vi "Main.vi"(11 "Module Admin":refnum<class "Delacor_lib_QMH_Module Admin.lvclass">) -> ()   [LabVIEW 2024, in "Explore.lvlib"]
doc: "This template is based off of the Queued Message Handler design pattern and the Queued Message Handler project template that ships with LabVIEW.\n\nThe main difference is that the queue is private to this module and communication between modules is performed via Broadcast and Request events.\n\nRequest events are wrapped in public API methods and are handled in the Event Handling Loop (EHL) of this VI. Any module can register for Broadcast events sent by this module. The EHL generates messages based on user interface actions.\n\nThe Message Handling Loop (MHL) processes messages generated by the EHL, or by other messages. The messages are string values, so new messages can be added easily to the Message Cases case structure in the MHL. Each message cluster can also provide an optional value for Message Data, which is a variant that can be converted to whatever message-specific data is required.\n_____\nBased on DQMH Project Template 7.0.1.1316."
uses:
  Explore.lvlib
  <vilib>/Delacor/Delacor QMH/Libraries/Module Admin_class/Delacor_lib_QMH_Module Admin.lvclass
  Module Data--cluster.ctl
  <vilib>/Delacor/Delacor QMH/Libraries/Message Queue_class/Delacor_lib_QMH_Message Queue.lvclass/Delacor_lib_QMH_Message Queue.ctl
  Stop Argument--cluster.ctl
  <vilib>/Delacor/Delacor QMH/Libraries/Module Admin_class/Delacor_lib_QMH_Module Admin.lvclass/Delacor_lib_QMH_Module Admin.ctl
  Update Table Argument--cluster.ctl
  Delete File Argument--cluster.ctl
  Get Reference Argument--cluster.ctl
  Get Reference (Reply Payload)--cluster.ctl
  <vilib>/Delacor/Delacor QMH/Libraries/Message Queue_class/Delacor_lib_QMH_Enqueue Message (Single).vi
  <vilib>/Delacor/Delacor QMH/Libraries/Module Admin_class/Delacor_lib_QMH_Get External Launch.vi
  <vilib>/Delacor/Delacor QMH/Libraries/Message Queue_class/Delacor_lib_QMH_Message Queue.lvclass
panel:
  in  "File List":i32(listbox)
  in  "Delete":bool
  out "error out":errorcluster
  out "Status":string
  in  "Simulate MHL Error":bool
  in  "Simulate EHL Error":bool
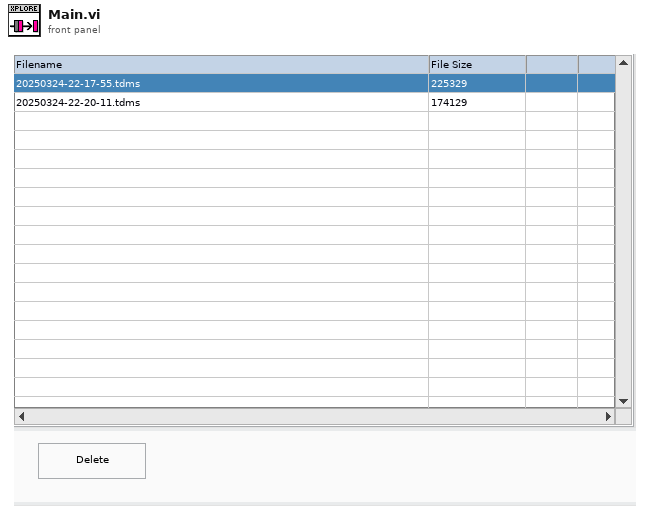
[diagram p1: front panel]
types:
  T1 = typedef "Explore.lvlib/Request Events--cluster.ctl" = cluster{"Stop Module":refnum<user-event>, "Show Panel":refnum<user-event>, "Hide Panel":refnum<user-event>, "Get Module Execution Status":refnum<user-event>, "Show Diagram":refnum<user-event>, "Update Table":refnum<user-event>, "Delete File":refnum<user-event>, "Get Reference":refnum<user-event>}
  T2 = typedef "Explore.lvlib/Module Data--cluster.ctl" = cluster{"Status":string, "Current Path":path}
  T3 = enum32{"invalid lock state", "Not Locked", "Locked (No Password)", "Password-protected"}
  T4 = typedef "Explore.lvlib/Stop Argument--cluster.ctl" = cluster{"Origin":string, "Exit via Stop Module Req?":bool, "Wait for Module to stop?":bool}
  T5 = typedef "Explore.lvlib/Update Table Argument--cluster.ctl" = cluster{"Log Folder":path}
  T6 = typedef "Explore.lvlib/Delete File Argument--cluster.ctl" = cluster{"File Name":string}
  T7 = typedef "Explore.lvlib/Get Reference Argument--cluster.ctl" = cluster{"Wait Notifier":refnum<notifier>, "wait for reply":bool}
  T8 = enum32{"Invalid", "Standard", "Closed", "Hidden", "Minimized", "Maximized"}
  T9 = typedef "Explore.lvlib/Get Reference (Reply Payload)--cluster.ctl" = cluster{"VI Refnum":refnum<vi>, "error":errorcluster}
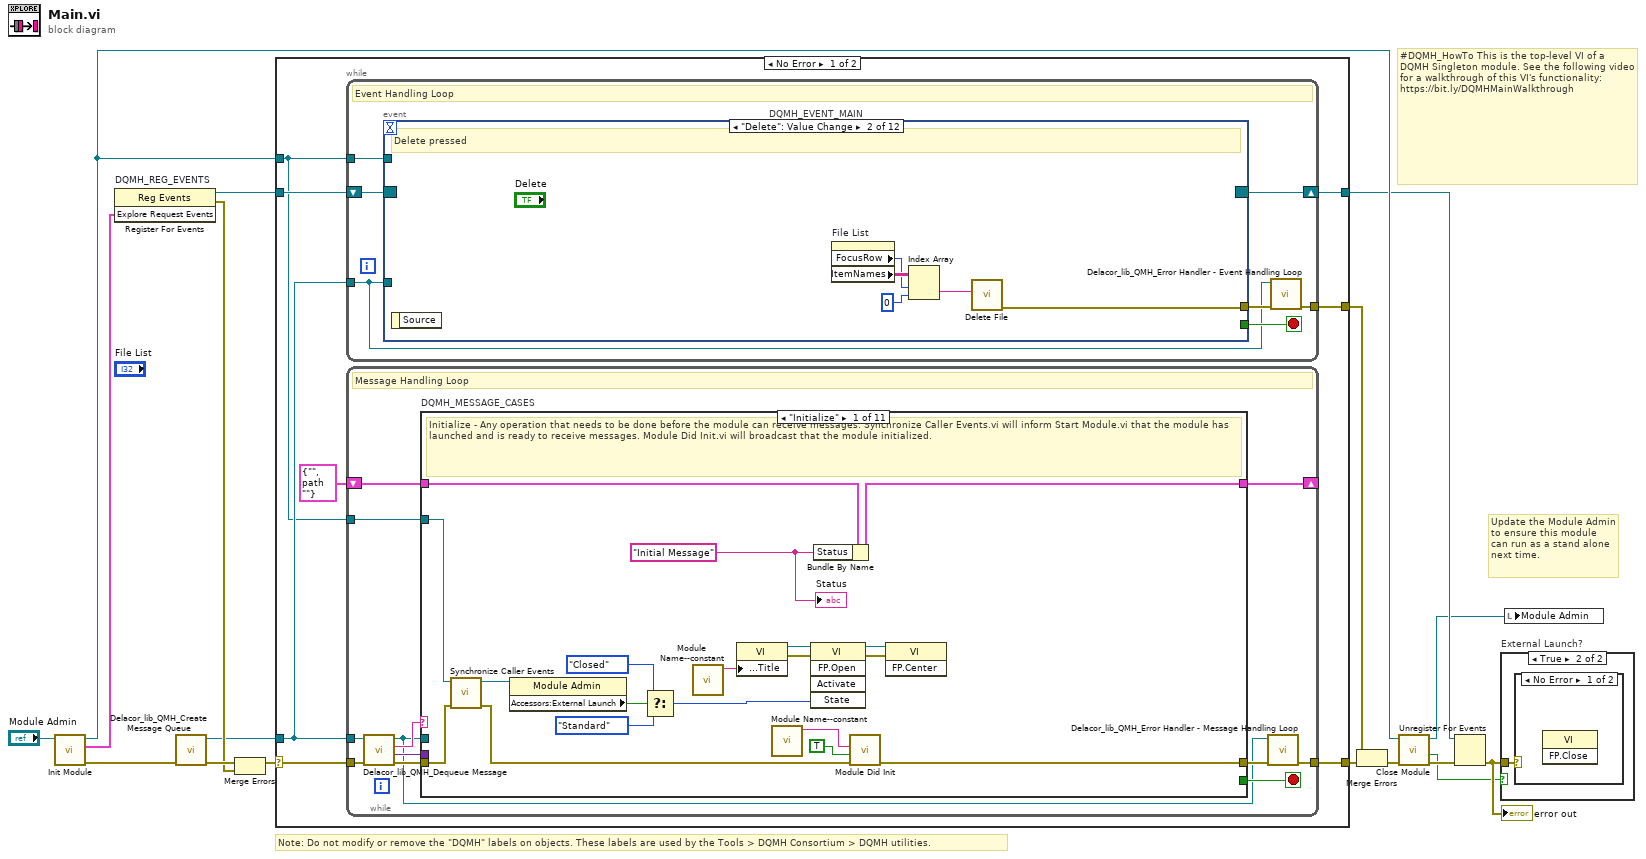
[diagram p0: block diagram]
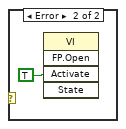
[diagram p3: hidden frame]
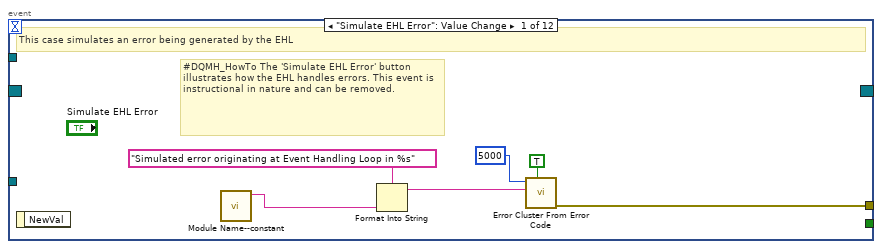
[diagram p4: hidden frame]
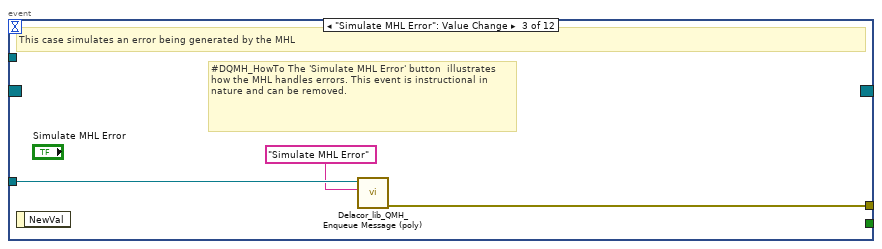
[diagram p5: hidden frame]
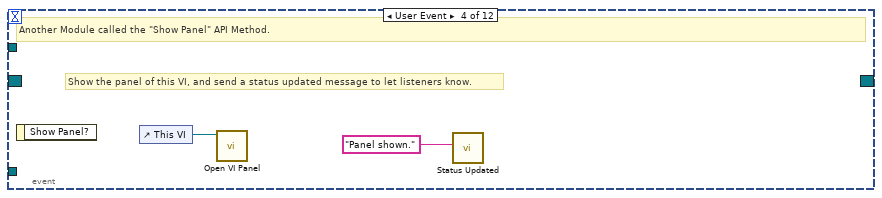
[diagram p6: hidden frame]
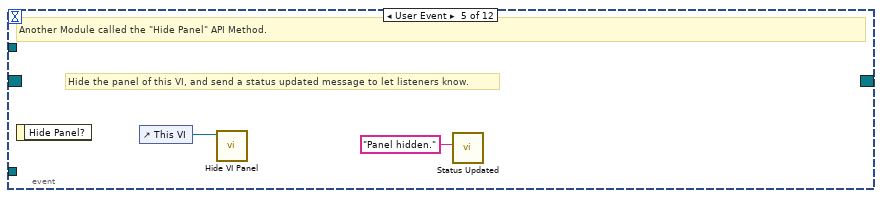
[diagram p7: hidden frame]
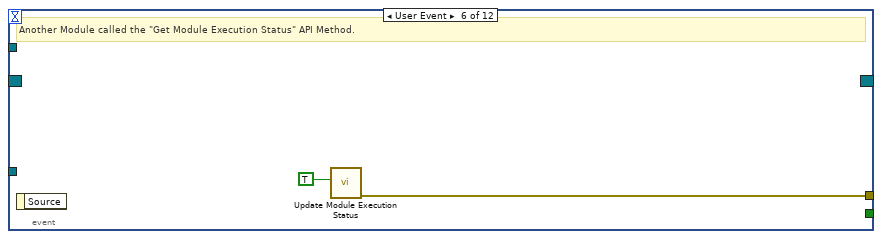
[diagram p8: hidden frame]
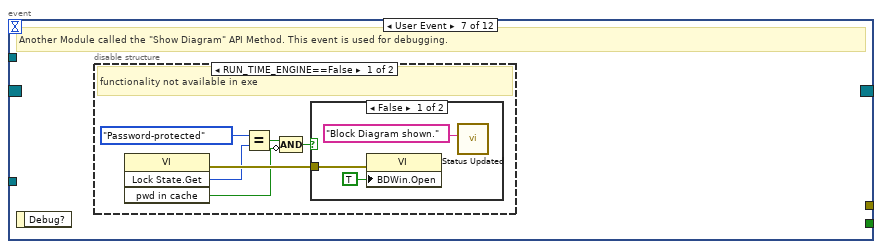
[diagram p9: hidden frame]
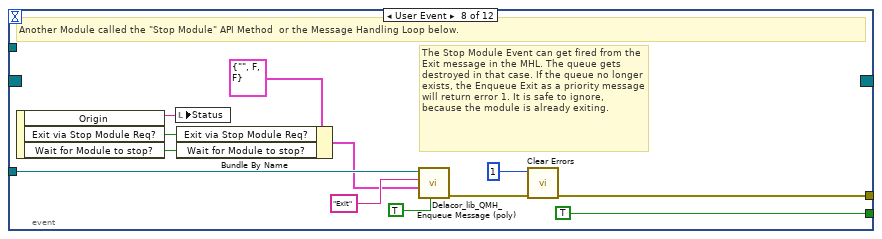
[diagram p12: hidden frame]
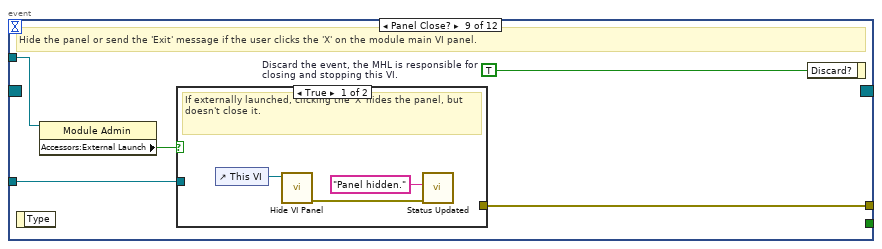
[diagram p13: hidden frame]
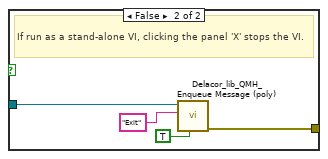
[diagram p14: hidden frame]
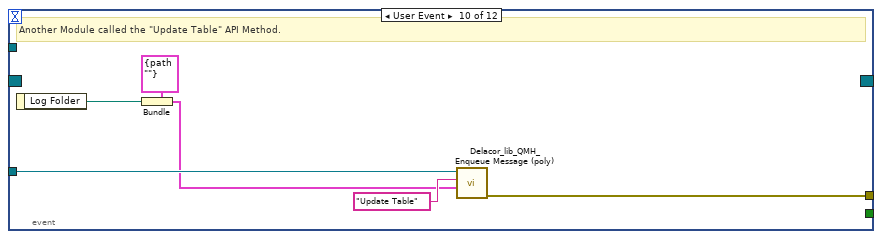
[diagram p15: hidden frame]
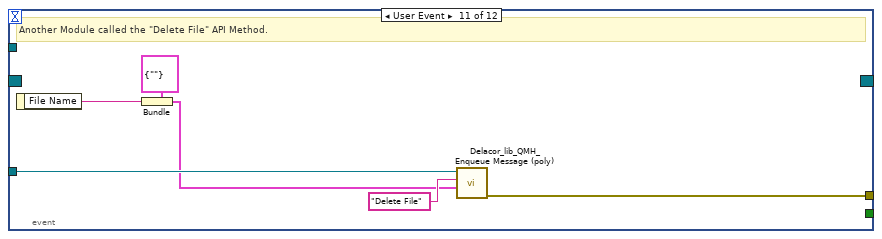
[diagram p16: hidden frame]
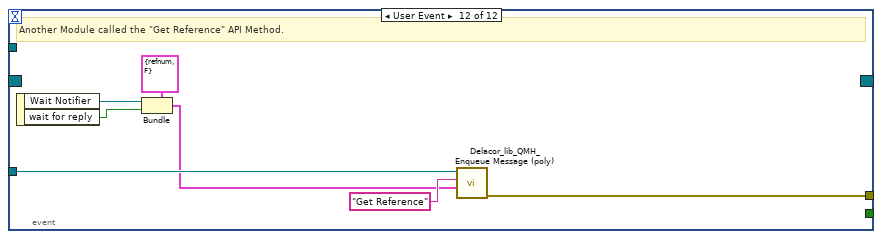
[diagram p17: hidden frame]
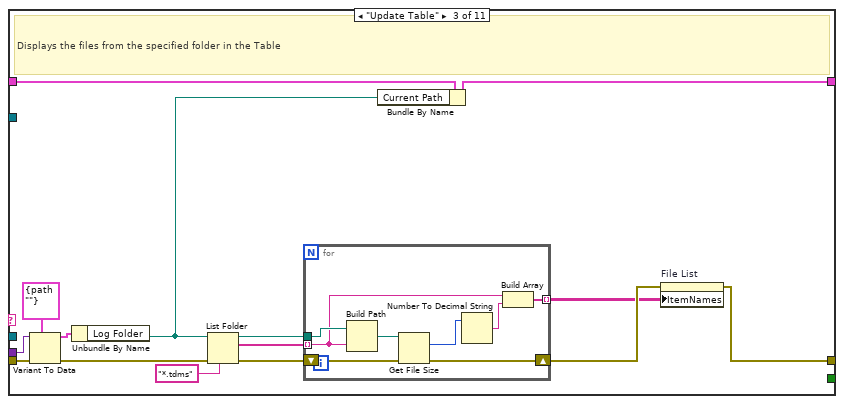
[diagram p19: hidden frame]
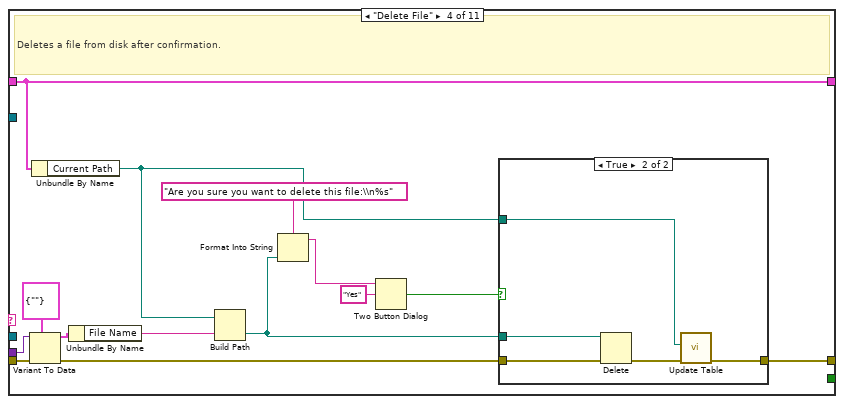
[diagram p20: hidden frame]
diagram:
  # "#DQMH_HowTo This is the top-level VI of a DQMH Singleton module. See the following video for a walkthrough of this VI's functionality: https://bit.ly/DQMHMainWalkthrough"
  # "Note: Do not modify or remove the \"DQMH\" labels on objects. These labels are used by the Tools > DQMH Consortium > DQMH utilities."
  # "Update the Module Admin to ensure this module can run as a stand alone next time."
  n1 = call "Init Module.vi"("Singleton Module Admin in"="Module Admin") -> ("error out"=w16:errorcluster, "Explore Request Events"=w5:T1, "Singleton Module Admin out"=w8:refnum<class "Delacor_lib_QMH_Module Admin.lvclass">)  [unwired: 8 in]
  n2 = register-events "DQMH_REG_EVENTS"(w5) -> (reference out=w6:refnum<event-registration>, error out=w9:errorcluster)  [unwired: 2 in]
  n3 = call <vilib>:"Delacor_lib_QMH_Create Message Queue.vi"("error in"=w16) -> ("error out"=w11:errorcluster, "Message Queue"=w4:refnum<class "Delacor_lib_QMH_Message Queue.lvclass">)  [unwired: 9 in]
  n4 = Merge Errors(w11, w9) -> (w10:errorcluster)
  n5 = case shown="No Error" w10 {
    selector: w10 -> [w23 w258]
    tunnel: [w25 w257] -> w17
    tunnel: [w22 w256] -> w7
    tunnel: w6 -> [w20 w256]
    tunnel: w4 -> [w19 w251]
    tunnel: [w24 _] -> w14
    tunnel: w8 -> [w18 w252]
    frame No Error {
      n6 = while {
        tunnel: w19 -> [w26]
        shift-right: [w29] -> w22
        shift-left: w20 -> [w30]
        tunnel: [w31] -> w24
        tunnel: w18 -> [w27]
        stop <- w28 stop-if-true
        # "Event Handling Loop"
        n7 = event "DQMH_EVENT_MAIN" shown="[1] \"Delete\": Value Change" {
          selector: w30 -> [_ _ _ _ _ _ _ _ _ _ _ _]
          dyn-events: [_ _ _ _ _ _ _ _ _ _ _ _] -> w29
          timeout: _ -> [_ _ _ _ _ _ _ _ _ _ _ _]
          tunnel: [_ _ _ _ _ _ _ TRUE ("Discard?") _ _ _ _] -> w28
          tunnel: w26 -> [_ _ w45 _ _ _ _ w69 w76 w91 w97 w104]
          tunnel: [w38 w43 w46 _ _ w52 _ w72 w78 w86 w92 w98] -> w32
          tunnel: w27 -> [_ _ _ _ _ _ _ _ w75 _ _ _]
          event "Simulate EHL Error": Value Change {
            # "#DQMH_HowTo The 'Simulate EHL Error' button  illustrates how the EHL handles errors. This event is instructional in nature and can be removed."
            # "This case simulates an error being generated by the EHL"
            n8 = event-data() -> ()  [unwired: 1 in, 1 out]
            n9 = call "Module Name--constant.vi"() -> ("Module Name"=w35:string)  [unwired: 11 in]
            n10 = Format Into String(format string="Simulated error originating at Event Handling Loop in %s", w35) -> (resulting string=w36:string)  [unwired: 2 in, 1 out]
            n11 = call <vilib>:"Error Cluster From Error Code.vi"("show call chain? (False)"=TRUE, "error message (\"\")"=w36, "error code (0)"=5000) -> ("error out"=w38:errorcluster)  [unwired: 6 in]
          }
          event "Delete": Value Change {
            # "Delete pressed"
            n12 = event-data() -> ()  [unwired: 1 in, 1 out]
            n13 = property on="File List" class="MCListbox (strict)"() -> ("FocusRow"=w40:i32, "ItemNames"=w42:string[][])  [unwired: 2 in, 2 out]
            n14 = Index Array(array=w42, index (row)=w40, index (col)=0 ("disabled index (col)")) -> (element=w39:string)
            n15 = call "Delete File.vi"("File Name"=w39) -> ("error out"=w43:errorcluster)  [unwired: 10 in]
          }
          event "Simulate MHL Error": Value Change {
            # "#DQMH_HowTo The 'Simulate MHL Error' button  illustrates how the MHL handles errors. This event is instructional in nature and can be removed."
            # "This case simulates an error being generated by the MHL"
            n16 = event-data() -> ()  [unwired: 1 in, 1 out]
            n17 = call-poly <vilib>:"Delacor_lib_QMH_Enqueue Message (poly).vi"("Message"="Simulate MHL Error", "Message Queue in"=w45) -> ("error out"=w46:errorcluster)  [unwired: 8 in, 1 out]
          }
          event User Event {
            # "Show the panel of this VI, and send a status updated message to let listeners know."
            # "Another Module called the \"Show Panel\" API Method."
            n18 = event-data() -> ()  [unwired: 1 in, 1 out]
            n19 = control-ref of="This VI"() -> (w48:refnum<vi>)
            n20 = call "Open VI Panel.vi"("VI"=w48) -> ()  [unwired: 10 in, 1 out]
            n21 = call "Status Updated.vi"("Status"="Panel shown." ("format string")) -> ()  [unwired: 10 in, 1 out]
          }
          event User Event {
            # "Hide the panel of this VI, and send a status updated message to let listeners know."
            # "Another Module called the \"Hide Panel\" API Method."
            n22 = event-data() -> ()  [unwired: 1 in, 1 out]
            n23 = control-ref of="This VI"() -> (w50:refnum<vi>)
            n24 = call "Hide VI Panel.vi"("VI"=w50) -> ()  [unwired: 10 in, 1 out]
            n25 = call "Status Updated.vi"("Status"="Panel hidden." ("format string")) -> ()  [unwired: 10 in, 1 out]
          }
          event User Event {
            # "Another Module called the \"Get Module Execution Status\" API Method."
            n26 = event-data() -> ()  [unwired: 1 in, 1 out]
            n27 = call "Update Module Execution Status.vi"("Running?"=TRUE) -> ("error out"=w52:errorcluster)  [unwired: 10 in]
          }
          event User Event {
            # "Another Module called the \"Show Diagram\" API Method. This event is used for debugging."
            n28 = event-data() -> ()  [unwired: 1 in, 1 out]
            n29 = disable-structure shown="RUN_TIME_ENGINE==False" {
              frame condition #0 (active) {
                # "functionality not available in exe"
                n30 = invoke on="Invoke Node" class="VI" method="Lock State.Get"() -> (error out=w58:errorcluster, "Get Lock State"=w57:T3, "pwd in cache"=w54:bool)  [unwired: 4 in, 1 out]
                n31 = Equal?(x=T3."Password-protected", y=w57) -> (x = y?=w55:bool)
                n32 = Compound Arithmetic op=AND(w55, invert w54) -> (w53:bool)
                n33 = case shown="False" w53 {
                  tunnel: w58 -> [w61 _]
                  frame False {
                    n34 = property on="Property Node" class="VI"(error in=w61, "BDWin.Open"=TRUE ("Block Diagram Window:Open")) -> ()  [unwired: 1 in, 2 out]
                    n35 = call "Status Updated.vi"("Status"="Block Diagram shown." ("format string")) -> ()  [unwired: 10 in, 1 out]
                  }
                  frame True {
                    # "Password-protected VI, and the password is not in the cache. Do not show the diagram."
                  }
                }
              }
              frame condition #1 {
              }
            }
          }
          event User Event {
            # "The Stop Module Event can get fired from the Exit message in the MHL. The queue gets destroyed in that case. If the queue no longer exists, the Enqueue Exit as a priority message will return error 1. It is safe to ignore, because the module is already exiting."
            # "Another Module called the \"Stop Module\" API Method  or the Message Handling Loop below."
            n36 = event-data() -> ("Origin"=w68:string, "Exit via Stop Module Req?"=w64:bool, "Wait for Module to stop?"=w63:bool)  [unwired: 1 in]
            n37 = local write "Status"(w68) -> ()
            n38 = Bundle By Name(cluster=T4 {"Origin"="", "Exit via Stop Module Req?"=FALSE, "Wait for Module to stop?"=FALSE} ("Stop Argument"), "Exit via Stop Module Req?"=w64, "Wait for Module to stop?"=w63) -> (w62:T4)
            n39 = call-poly <vilib>:"Delacor_lib_QMH_Enqueue Message (poly).vi"("Priority Message? (F)"=TRUE, "Message Data"=w62, "Message"="Exit", "Message Queue in"=w69) -> ("error out"=w73:errorcluster)  [unwired: 6 in, 1 out]
            n40 = call <vilib>:"Clear Errors.vi"("error in (no error)"=w73, "specific error code to clear (0: all)"=1) -> ("error out"=w72:errorcluster)  [unwired: 4 in, 1 out]
          }
          event Panel Close? {
            w77 = TRUE  # Discard the event, the MHL is responsible for closing and stopping this VI.
            # "Hide the panel or send the 'Exit' message if the user clicks the 'X' on the module main VI panel."
            n41 = event-data() -> ()  [unwired: 1 in, 1 out]
            n42 = property on="Property Node" class="Module Admin"(reference=w75) -> ("Accessors:External Launch"=w74:bool)  [unwired: 1 in, 2 out]
            n43 = case shown="True" w74 {
              tunnel: w76 -> [_ w84]
              tunnel: [_ w85] -> w78
              frame True {
                # "If externally launched, clicking the 'X' hides the panel, but doesn't close it."
                n44 = control-ref of="This VI"() -> (w81:refnum<vi>)
                n45 = call "Hide VI Panel.vi"("VI"=w81) -> ("error out"=w79:errorcluster)  [unwired: 10 in]
                n46 = call "Status Updated.vi"("error in"=w79, "Status"="Panel hidden." ("format string")) -> ()  [unwired: 9 in, 1 out]
              }
              frame False {
                # "If run as a stand-alone VI, clicking the panel 'X' stops the VI."
                n47 = call-poly <vilib>:"Delacor_lib_QMH_Enqueue Message (poly).vi"("Priority Message? (F)"=TRUE, "Message"="Exit", "Message Queue in"=w84) -> ("error out"=w85:errorcluster)  [unwired: 7 in, 1 out]
              }
            }
            n48 = event-data ("Event Filter Node")("Discard?"=w77) -> ()  [unwired: 1 in, 1 out]
          }
          event User Event {
            # "Another Module called the \"Update Table\" API Method."
            n49 = event-data() -> ("Log Folder"=w87:path)  [unwired: 1 in]
            n50 = Bundle(cluster=T5 {"Log Folder"=path ""} ("Update Table Argument"), "Log Folder"=w87) -> (w88:T5)
            n51 = call-poly <vilib>:"Delacor_lib_QMH_Enqueue Message (poly).vi"("Message Data"=w88, "Message"="Update Table", "Message Queue in"=w91) -> ("error out"=w86:errorcluster)  [unwired: 7 in, 1 out]
          }
          event User Event {
            # "Another Module called the \"Delete File\" API Method."
            n52 = event-data() -> ("File Name"=w93:string)  [unwired: 1 in]
            n53 = Bundle(cluster=T6 {"File Name"=""} ("Delete File Argument"), "File Name"=w93) -> (w94:T6)
            n54 = call-poly <vilib>:"Delacor_lib_QMH_Enqueue Message (poly).vi"("Message Data"=w94, "Message"="Delete File", "Message Queue in"=w97) -> ("error out"=w92:errorcluster)  [unwired: 7 in, 1 out]
          }
          event User Event {
            # "Another Module called the \"Get Reference\" API Method."
            n55 = event-data() -> ("Wait Notifier"=w100:refnum<notifier>, "wait for reply"=w99:bool)  [unwired: 1 in]
            n56 = Bundle(cluster=T7 {"Wait Notifier"=refnum, "wait for reply"=FALSE} ("Get Reference Argument"), "Wait Notifier"=w100, "wait for reply"=w99) -> (w101:T7)
            n57 = call-poly <vilib>:"Delacor_lib_QMH_Enqueue Message (poly).vi"("Message Data"=w101, "Message"="Get Reference", "Message Queue in"=w104) -> ("error out"=w98:errorcluster)  [unwired: 7 in, 1 out]
          }
        }
        n58 = call-dynamic "Delacor_lib_QMH_Error Handler - Event Handling Loop.vi"("error in"=w32, "Message Queue in"=w26) -> ("dup error in"=w31:errorcluster)  [unwired: 8 in, 1 out]
      }
      n59 = while {
        tunnel: w19 -> [w105]
        shift-right: [w113] -> _
        shift-left: T2 {"Status"="", "Current Path"=path ""} ("Data Cluster") -> [w114]
        tunnel: w23 -> [w116]
        tunnel: [w108] -> w25
        tunnel: w18 -> [w109]
        stop <- w112 stop-if-true
        # "Message Handling Loop"
        n60 = call-dynamic "Delacor_lib_QMH_Dequeue Message.vi"("error in"=w116, "Message Queue in"=w105) -> ("error out"=w115:errorcluster, "Message Data"=w110:variant, "Message"=w111:string, "Message Queue out"=w106:refnum<class "Delacor_lib_QMH_Message Queue.lvclass">)  [unwired: 6 in]
        n61 = case "DQMH_MESSAGE_CASES" shown="\"Initialize\"" w111 {
          selector: w111 -> [_ _ _ _ _ _ _ _ _ _ w246]
          tunnel: w106 -> [_ _ _ _ _ _ _ _ w212 w234 _]
          tunnel: w115 -> [w133 w137 w152 w174 w192 w197 w199 w208 w219 w240 w249]
          tunnel: [w131 w137 w141 w166 w182 w196 w199 w207 w215 w235 w250] -> w107
          tunnel: w114 -> [w122 w136 w151 w163 w191 w195 w198 w205 w214 w233 w247]
          tunnel: [w121 w136 w139 w163 w191 w195 w198 w205 w214 w233 w247] -> w113
          tunnel: [_ _ _ _ _ _ _ _ _ w232 _] -> w112
          tunnel: w110 -> [_ _ w149 w172 w189 _ _ _ w213 w231 _]
          tunnel: w109 -> [w123 _ _ _ _ _ _ _ w211 w226 _]
          frame "Initialize" {
            w117 = "Initial Message" ("Initial Message")
            # "Initialize - Any operation that needs to be done before the module can receive messages. Synchronize Caller Events.vi will inform Start Module.vi that the module has launched and is ready to receive messages. Module Did Init.vi will broadcast that the module initialized."
            n62 = call "Synchronize Caller Events.vi"("error in"=w133, "Singleton Module Admin in"=w123) -> ("error out"=w132:errorcluster, "Singleton Module Admin out"=w118:refnum<class "Delacor_lib_QMH_Module Admin.lvclass">)  [unwired: 8 in]
            n63 = property on="Property Node" class="Module Admin"(reference=w118) -> ("Accessors:External Launch"=w127:bool)  [unwired: 1 in, 2 out]
            n64 = Select(t=T8."Closed" ("State"), s=w127, f=T8."Standard" ("State")) -> (s? t:f=w124:T8)
            n65 = call "Module Name--constant.vi"() -> ("Module Name"=w130:string)  [unwired: 11 in]
            n66 = property on="Property Node" class="VI"("Front Panel.Title"=w130) -> (reference out=w129:refnum<vi>, error out=w135:errorcluster)  [unwired: 2 in]
            n67 = call "Module Name--constant.vi"() -> ("Module Name"=w119:string)  [unwired: 11 in]
            n68 = invoke on="Invoke Node" class="VI" method="FP.Open"(reference=w129, error in=w135, "State"=w124) -> (reference out=w128:refnum<vi>, error out=w134:errorcluster)  [unwired: 2 in, 3 out]
            n69 = Bundle By Name(cluster=w122, "Status"=w117) -> (w121:T2)
            n70 = call "Module Did Init.vi"("error in"=w132, "Initialized?"=TRUE, "Origin"=w119) -> ("error out"=w131:errorcluster)  [unwired: 8 in]
            n71 = invoke on="Invoke Node" class="VI" method="FP.Center"(reference=w128, error in=w134) -> ()  [unwired: 1 in, 3 out]
            "Status" <- w117
          }
          frame "---Module Specific---" {
            # "Separator -- The following cases handle messages specific to this Module."
          }
          frame "Update Table" {
            # "Displays the files from the specified folder in the Table"
            n72 = Variant To Data(error in=w152, type=T5 {"Log Folder"=path ""} ("Update Table Argument"), Variant=w149) -> (data=w147:T5, error out=w150:errorcluster)
            n73 = Unbundle By Name(w147) -> ("Log Folder"=w138:path)
            n74 = List Folder(path=w138, pattern="*.tdms", error in=w150) -> (path out=w143:path, filenames=w144:string[], error out=w145:errorcluster)  [unwired: 1 in, 1 out]
            n75 = for {
              shift-right: [w159] -> w142
              shift-left: w145 -> [w160]
              tunnel: w144 -> [w154] mode=indexing
              tunnel: w143 -> [w158]
              tunnel: [w153] -> w140 mode=indexing
              n76 = Build Path(base path=w158, name or relative path=w154) -> (appended path=w157:path)
              n77 = Get File Size(file=w157, error in=w160) -> (size (in bytes)=w156:i64, 0:w159:errorcluster)  [unwired: 1 out]
              n78 = Number To Decimal String(number=w156) -> (decimal integer string=w155:string)  [unwired: 1 in]
              n79 = Build Array(w154, w155) -> (w153:string[])
            }
            n80 = Bundle By Name(cluster=w151, "Current Path"=w138) -> (w139:T2)
            n81 = property on="File List" class="MCListbox (strict)"(error in=w142, "ItemNames"=w140) -> (error out=w141:errorcluster)  [unwired: 1 in, 1 out]
          }
          frame "Delete File" {
            # "Deletes a file from disk after confirmation."
            n82 = Variant To Data(error in=w174, type=T6 {"File Name"=""} ("Delete File Argument"), Variant=w172) -> (data=w170:T6, error out=w173:errorcluster)
            n83 = Unbundle By Name(w163) -> ("Current Path"=w161:path)
            n84 = Unbundle By Name(w170) -> ("File Name"=w164:string)
            n85 = Build Path(base path=w161, name or relative path=w164) -> (appended path=w162:path)
            n86 = Format Into String(format string="Are you sure you want to delete this file:\\n%s", w162) -> (resulting string=w168:string)  [unwired: 2 in, 1 out]
            n87 = Two Button Dialog(message=w168, 2:"Yes" ("T button name (\"OK\")")) -> (T button?=w165:bool)  [unwired: 1 in]
            n88 = case shown="True" w165 {
              tunnel: w173 -> [w175 w180]
              tunnel: [w175 w177] -> w166
              tunnel: w162 -> [_ w178]
              tunnel: w161 -> [_ w176]
              frame False {
              }
              frame True {
                n89 = Delete(path (use dialog)=w178, error in=w180) -> (error out=w179:errorcluster)  [unwired: 3 in, 2 out]
                n90 = call "Update Table.vi"("error in"=w179, "Log Folder"=w176) -> ("error out"=w177:errorcluster)  [unwired: 9 in]
              }
            }
          }
          frame "Get Reference" {
            # "Returns the main.vi reference to insert into a subpanel in a calling VI."
            n91 = Variant To Data(error in=w192, type=T7 {"Wait Notifier"=refnum, "wait for reply"=FALSE} ("Get Reference Argument"), Variant=w189) -> (data=w187:T7, error out=w190:errorcluster)
            n92 = Unbundle By Name(w187) -> ("Wait Notifier"=w186:refnum<notifier>, "wait for reply"=w185:bool)
            n93 = control-ref of="This VI"() -> (w181:refnum<vi>)
            n94 = Bundle By Name(cluster=T9 {"VI Refnum"=refnum, "error"={"status"=FALSE, "code"=0, "source"=""}} ("Get Reference (Reply Payload)"), "VI Refnum"=w181) -> (w184:T9)
            n95 = Merge Errors(w190) -> (w182:errorcluster)
            n96 = case "DQMH_FIRE_NOTIFIER" shown="True" w185 {
              tunnel: w186 -> [_ w194]
              tunnel: w184 -> [_ w193]
              frame False {
              }
              frame True {
                n97 = Send Notification(notification=w193, notifier=w194) -> ()  [unwired: 1 in, 2 out]
              }
            }
          }
          frame "---Copy This Frame---" {
            # "Duplicate this frame when creating new messages.  Change this comment in the duplicated frame to describe this message."
            n98 = Merge Errors(w197) -> (w196:errorcluster)
          }
          frame "---Exit and Error Handling---" {
            # "Separator - The following cases handle errors and exit messages."
          }
          frame "Simulate MHL Error" {
            # "#DQMH_HowTo The 'Simulate MHL Error' button  illustrates how the MHL handles errors. This event is instructional in nature and can be removed."
            # "Simulate an error occurring at the MHL"
            n99 = call "Module Name--constant.vi"() -> ("Module Name"=w201:string)  [unwired: 11 in]
            n100 = Format Into String(format string="Simulated error originating at Message Handling Loop in %s", w201) -> (resulting string=w202:string)  [unwired: 2 in, 1 out]
            n101 = call <vilib>:"Error Cluster From Error Code.vi"("show call chain? (False)"=TRUE, "error message (\"\")"=w202, "error code (0)"=5001) -> ("error out"=w206:errorcluster)  [unwired: 6 in]
            n102 = Merge Errors(w208, w206) -> (w207:errorcluster)
          }
          frame "Error" {
            # "#CodeRecommended - If the module is running in standalone mode (External Launch = FALSE), this code will pop up an error dialog and call the 'Exit' message if an error occurs. Add more fine-grained error management here."
            # "Error - Check the error message data and respond accordingly. This message is sent by the \"Error Handler\" VIs at the end of each loop in this application."
            n103 = property on="Property Node" class="Module Admin"(reference=w211) -> ("Accessors:External Launch"=w210:bool)  [unwired: 1 in, 2 out]
            n104 = Variant To Data(error in=w219, type=errorcluster {"status"=FALSE, "code"=0, "source"=""} ("error constant"), Variant=w213) -> (data=w209:errorcluster, error out=w217:errorcluster)
            n105 = local write "error out"(w209) -> ()
            n106 = call "Error Reported.vi"("Error"=w209) -> ()  [unwired: 10 in, 1 out]
            n107 = case shown="False" w210 {
              tunnel: [w224 _] -> w216
              tunnel: w212 -> [w222 _]
              tunnel: w209 -> [w223 _]
              frame False {
                n108 = disable-structure shown="Default" {
                  disable-tunnel: w223 -> [w225 _]
                  frame condition #0 (active) {
                    # "If the module is running standalone, then pop up an error dialog and call the \"Exit\" message."
                    n109 = call <vilib>:"Simple Error Handler.vi"("error in (no error)"=w225) -> ()  [unwired: 4 in, 5 out]
                  }
                  frame condition #1 {
                    # "To prevent the Simple Error Handler VI from being loaded (e.g. when deploying to a Real-Time target), add the Conditional Disable Symbol \"DQMH_Disable_SEH\" to your project and set it to TRUE."
                  }
                }
                n110 = call-poly <vilib>:"Delacor_lib_QMH_Enqueue Message (poly).vi"("Priority Message? (F)"=TRUE, "Message"="Exit", "Message Queue in"=w222) -> ("error out"=w224:errorcluster)  [unwired: 7 in, 1 out]
              }
              frame True {
                # "If the module was launched externally, calling the Error Reported broadcast VI is the only action performed by the \"Error\" message. The module's caller can then process the error appropriately."
              }
            }
            n111 = Merge Errors(w217, w216) -> (w215:errorcluster)
          }
          frame "Exit" {
            w230 = 91  # 91: not all Exit messages will have an argument
            w232 = TRUE  # Stop the VI
            # "Release the message queue reference"
            # "#CodeNeeded - Add any required cleanup code here."
            # "Exit - Exit the application."
            n112 = Variant To Data(error in=w240, type=T4 {"Origin"="", "Exit via Stop Module Req?"=FALSE, "Wait for Module to stop?"=FALSE} ("Stop Argument"), Variant=w231) -> (data=w228:T4, error out=w237:errorcluster)
            n113 = call <vilib>:"Clear Errors.vi"("error in (no error)"=w237, "specific error code to clear (0: all)"=w230) -> ("error out"=w239:errorcluster)  [unwired: 4 in, 1 out]
            n114 = control-ref of="This VI"() -> (w227:refnum<vi>)
            n115 = call-dynamic "Delacor_lib_QMH_Release Message Queue.vi"("error in"=w239, "Message Queue"=w234) -> ("error out"=w238:errorcluster)  [unwired: 9 in]
            n116 = call "Handle Exit.vi"("Stop Argument"=w228, "Admin in"=w226, "VI reference"=w227) -> ("error out"=w236:errorcluster)  [unwired: 7 in, 1 out]
            n117 = Merge Errors(w238, w236) -> (w235:errorcluster)
            n118 = call "Error Reported.vi"("Error"=w235) -> ()  [unwired: 10 in, 1 out]
          }
          frame Default {
            # "'Default' case only runs if there is a message that isn't defined in any of the other cases.  Output a programming error."
            n119 = call "Module Name--constant.vi"() -> ("Module Name"=w245:string)  [unwired: 11 in]
            n120 = Format Into String(format string="The invalid message string \"%s\" was received in the Message Handling Loop for module \"%s\".", w246, w245) -> (resulting string=w241:string)  [unwired: 2 in, 1 out]
            n121 = call <vilib>:"Error Cluster From Error Code.vi"("show call chain? (False)"=TRUE, "error message (\"\")"=w241, "error code (0)"=1) -> ("error out"=w248:errorcluster)  [unwired: 6 in]
            n122 = Merge Errors(w249, w248) -> (w250:errorcluster)
          }
        }
        n123 = call-dynamic "Delacor_lib_QMH_Error Handler - Message Handling Loop.vi"("error in"=w107, "Message Queue in"=w106) -> ("dup error in"=w108:errorcluster)  [unwired: 8 in, 1 out]
      }
    }
    frame Error {
      # "Synchronize Caller Events.vi will inform Start Module.vi that the module has launched and will let the code calling Start Module.vi register for broadcasts and would permit the caller receive the broadcast that an error occurred at launch time."
      n124 = call-dynamic "Delacor_lib_QMH_Release Message Queue.vi"("error in"=w258, "Message Queue"=w251) -> ("error out"=w257:errorcluster)  [unwired: 9 in]
      n125 = call "Synchronize Caller Events.vi"("Singleton Module Admin in"=w252) -> ("error out"=w259:errorcluster)  [unwired: 9 in, 1 out]
      n126 = call "Module Name--constant.vi"() -> ("Module Name"=w255:string)  [unwired: 11 in]
      n127 = Format Into String(format string="An error occurred during initialization. %s is no longer running.", w255) -> (resulting string=w253:string)  [unwired: 2 in, 1 out]
      n128 = Merge Errors(w257, w259) -> (w260:errorcluster)
      n129 = call "Error Reported.vi"("Additional Information"=w253, "Error"=w260) -> ()  [unwired: 9 in, 1 out]
    }
  }
  n130 = Merge Errors(w14, w17) -> (w13:errorcluster)
  n131 = call "Close Module.vi"("error in"=w13, "Module Admin in"=w8) -> ("error out"=w15:errorcluster, "External Launch"=w1:bool, "Module Admin out"=w2:refnum<class "Delacor_lib_QMH_Module Admin.lvclass">)  [unwired: 7 in]
  n132 = Unregister For Events(event registration refnum=w7, error in=w15) -> (error out=w12:errorcluster)
  "error out" <- w12
  n133 = case "External Launch?" shown="True" w1 {
    tunnel: w12 -> [_ w261]
    frame False {
    }
    frame True {
      n134 = case shown="No Error" w261 {
        frame No Error {
          n135 = invoke on="Invoke Node" class="VI" method="FP.Close"() -> ()  [unwired: 3 in, 3 out]
        }
        frame Error {
          n136 = invoke on="Invoke Node" class="VI" method="FP.Open"("Activate"=TRUE ("Activate?")) -> ()  [unwired: 4 in, 5 out]
        }
      }
    }
  }
  n137 = local write "Module Admin"(w2) -> ()
